vi "IsSatisfied.vi"(10 "Product":refnum<class "Product.lvclass">, 11 "SizeSpecification":refnum<class "SizeSpecification.lvclass">) -> (2 "IsSatisfied":bool)   [LabVIEW 2018, in "SizeSpecification.lvclass"]
uses:
  SizeSpecification.lvclass
  Product/Product.lvclass
  SizeSpecification.lvclass/SizeSpecification.ctl
  Product/Product.lvclass/Product.ctl
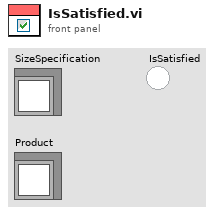
[diagram p1: front panel]
types:
  T1 = typedef "Product.lvclass/Size.ctl" = enum16{"Yuge", "Big", "Medium", "Small"}
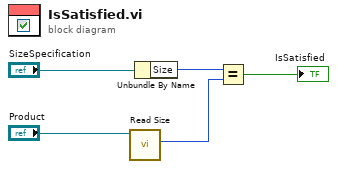
[diagram p0: block diagram]
diagram:
  n1 = call "Read Size.vi"("Product In"="Product") -> ("Size"=w3:T1)  [unwired: 9 in, 1 out]
  n2 = Unbundle By Name("SizeSpecification") -> ("Size"=w2:T1)
  n3 = Equal?(x=w2, y=w3) -> (x = y?=→"IsSatisfied":bool)
